vi "ReadingDebuggingMessages.vi"() -> ()   [LabVIEW 2014]
uses:
  RTI/GIT_HEAD/connextdds/lvdds.1.0/srcLV/lvdds.1.0_package/Library/LVDDS_library.lvlib
panel:
  in  "stop":bool
  out "Debugging table":string[][](table)
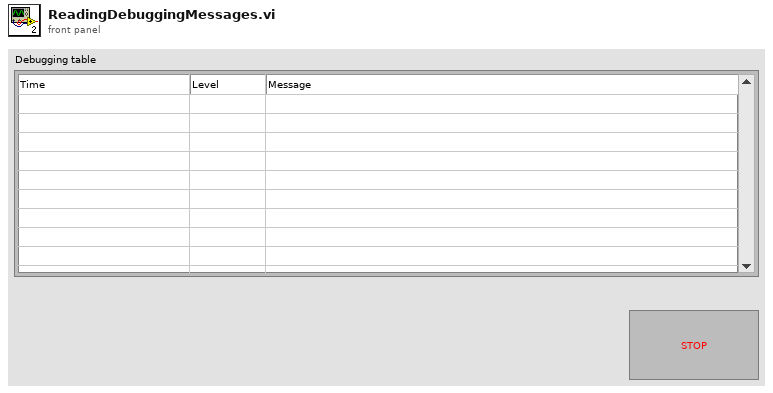
[diagram p1: front panel]
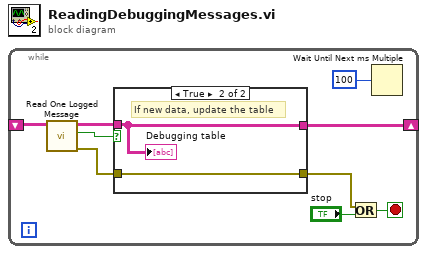
[diagram p0: block diagram]
diagram:
  n1 = while {
    shift-right: [w4] -> _
    shift-left: _ -> [w3]
    stop <- w9 stop-if-true
    n2 = call "Read One Logged Message.vi"("Debugging table in"=w3) -> ("Debugging table out"=w6:string[][], "Print table?"=w7:bool, "error out"=w5:errorcluster)  [unwired: 7 in]
    n3 = case shown="True" w7 {
      tunnel: w6 -> [w10 w13]
      tunnel: w5 -> [w11 w12]
      tunnel: [w11 w12] -> w1
      tunnel: [w10 w13] -> w4
      frame False {
      }
      frame True {
        # "If new data, update the table"
        "Debugging table" <- w13
      }
    }
    n4 = Or(x=w1, y="stop") -> (x .or. y?=w9:bool)
    n5 = Wait Until Next ms Multiple(millisecond multiple=u32 100) -> ()  [unwired: 1 out]
  }
